vi "Read counter.vi"(8 "error in (no error)":errorcluster, 11 "Counter name (dflt=blank)":string) -> (0 "error out":errorcluster, 3 "Value":i32)   [LabVIEW 2021, in "Named Counters.lvlib"]
uses:
  Named Counters.lvlib
  Counter global variable.vi
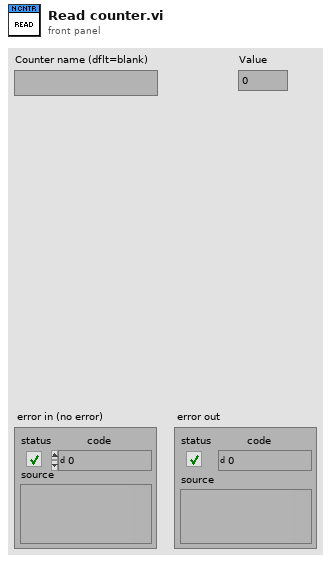
[diagram p1: front panel]
types:
  T1 = typedef "Named Counters.lvlib/Counter Cluster.ctl" = cluster{"Name":string, "Value":i32}
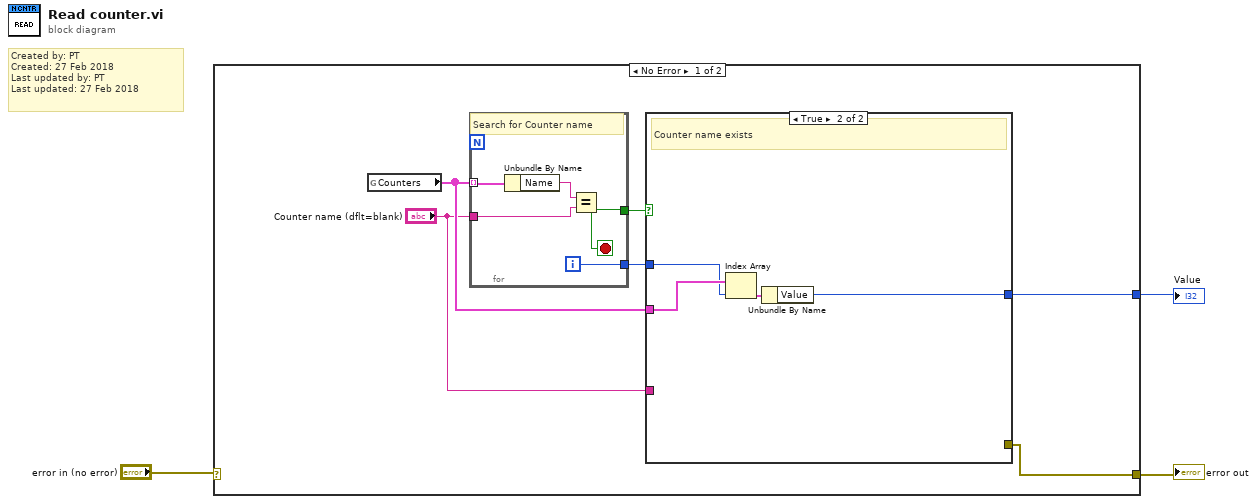
[diagram p0: block diagram]
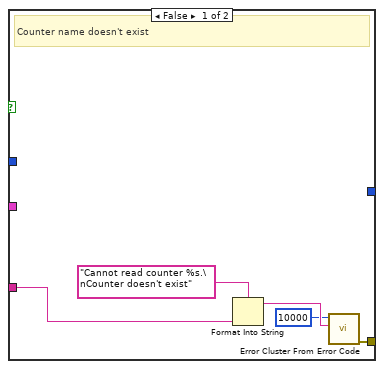
[diagram p2: hidden frame]
diagram:
  # "Created by: PT\nCreated: 27 Feb 2018\nLast updated by: PT\nLast updated: 27 Feb 2018"
  n1 = case shown="No Error" "error in (no error)" {
    selector: "error in (no error)" -> [_ w24]
    tunnel: [w4 w24] -> w2
    tunnel: [w5 _] -> w1
    frame No Error {
      n2 = global read "Counter global variable.vi" "Counters"() -> (w8:T1[])
      n3 = for {
        tunnel: w8 -> [w23] mode=indexing
        tunnel: "Counter name (dflt=blank)" -> [w21]
        tunnel: [w20] -> w9
        tunnel: [w19] -> w6
        i -> [w19]
        stop <- w20 stop-if-true
        # "Search for Counter name"
        n4 = Unbundle By Name(w23) -> ("Name"=w22:string)
        n5 = Equal?(x=w22, y=w21) -> (x = y?=w20:bool)
      }
      n6 = case shown="True" w9 {
        tunnel: w8 -> [_ w18]
        tunnel: "Counter name (dflt=blank)" -> [w10 _]
        tunnel: w6 -> [_ w17]
        tunnel: [_ w15] -> w5
        tunnel: [w11 _] -> w4
        frame False {
          # "Counter name doesn't exist"
          n7 = Format Into String(format string="Cannot read counter %s.\nCounter doesn't exist" ("error message (\"\")"), w10) -> (resulting string=w14:string)  [unwired: 2 in, 1 out]
          n8 = call <vilib>:"Error Cluster From Error Code.vi"("error message (\"\")"=w14, "error code (0)"=10000) -> ("error out"=w11:errorcluster)  [unwired: 7 in]
        }
        frame True {
          # "Counter name exists"
          n9 = Index Array(array=w18, index=w17) -> (element=w16:T1)
          n10 = Unbundle By Name(w16) -> ("Value"=w15:i32)
        }
      }
    }
    frame Error {
    }
  }
  "error out" <- w2
  "Value" <- w1
